vi "JKI-JSON Test Marshall-Unmarshall.vi"() -> ()   [LabVIEW 2019]
uses:
  Test Cluster.ctl
  <vilib>/addons/_JKI.lib/Serialization/JSON/Library/Timestamp Options.ctl
  source/Serializer.JSON.lvclass
  C:/Program Files (x86)/National Instruments/LabVIEW 2019/vi.lib/LabVIEW Open Source Project/OpenSerializer/Serializer/Serializer.lvclass
  source/Serializer.JSON.lvclass/Serializer.JSON.ctl
  source/Write Enums As String.vi
  source/Write Multiline.vi
  source/Write Numeric Extensions.vi
  source/Write Timestamp Options.vi
  <vilib>/LabVIEW Open Source Project/OpenSerializer/Serializer/Serializer.lvclass
  <vilib>/addons/_JKI.lib/Serialization/JSON/JKI JSON Serialization.lvlib
panel:
  in  "Timestamp Options":T1={"Convert Timestamps"=TRUE, "UTC"=FALSE}
  in  "Numeric Extensions":bool=TRUE
  in  "Multiline":bool=TRUE
  in  "Enums As String":bool=TRUE
  out "error out":errorcluster
  out "Pass?":bool
  out "Data Cluster out":T2={"Top-Level"={"Boolean"=FALSE, "String"="", "Path"=path "", "Numeric"=0.0, "Enum"=enum."Item0", "Array"=[], "Sub-Cluster"={"Numeric"=0.0, "Boolean"=FALSE, "Empty String"=""}, "Multi-Line String"=""}} {"Top-Level"."Numeric" format="%#_10g"}
  out "JSON String":string
  in  "Data Cluster in":T2={"Top-Level"={"Boolean"=FALSE, "String"="Another test string", "Path"=path "C:/Windows", "Numeric"=4.0, "Enum"=enum."Item0", "Array"=[0.0, 1.0, 2.0, 3.0, 4.0, 5.0, 6.0], "Sub-Cluster"={"Numeric"=0.0, "Boolean"=TRUE, "Empty String"="Test String Here"}, "Multi-Line String"="Test String Here\nLine2\nLine3"}} {"Top-Level"."Numeric" format="%#_10g"}
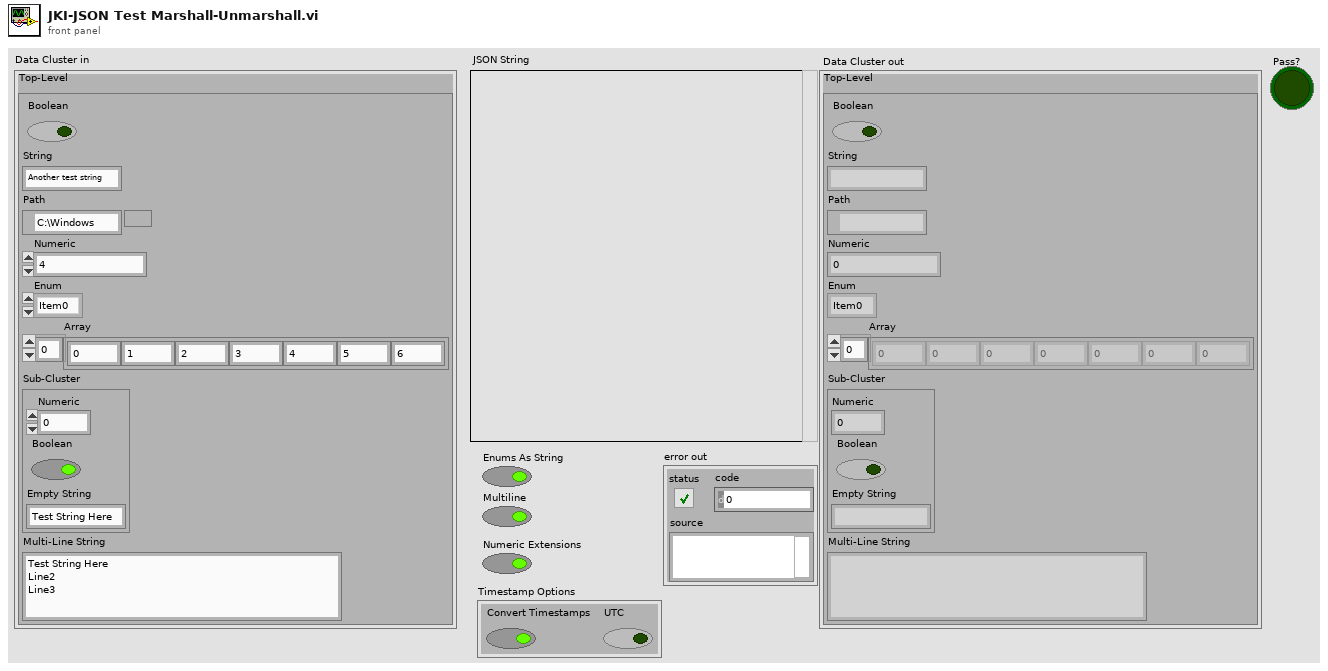
[diagram p1: front panel]
types:
  T1 = typedef "JKI JSON Serialization.lvlib/Timestamp Options.ctl" = cluster{"Convert Timestamps":bool, "UTC":bool}
  T2 = typedef "Test Cluster.ctl" = cluster{"Top-Level":cluster{"Boolean":bool, "String":string, "Path":path, "Numeric":dbl, "Enum":enum16{"Item0", "Item1"}, "Array":dbl[], "Sub-Cluster":cluster{"Numeric":dbl, "Boolean":bool, "Empty String":string}, "Multi-Line String":string}}
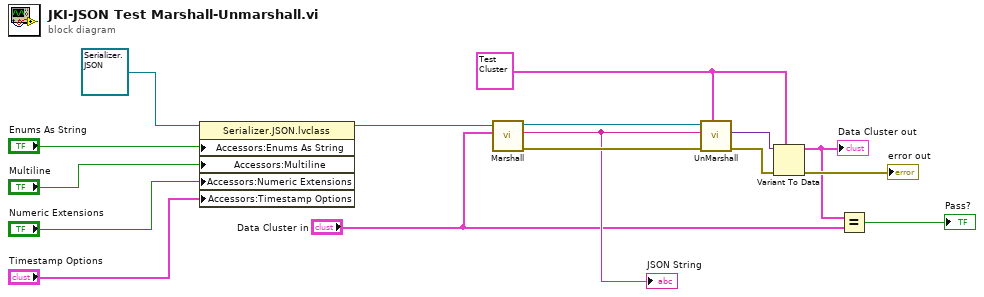
[diagram p0: block diagram]
diagram:
  w12 = T2 {"Top-Level"={"Boolean"=FALSE, "String"="", "Path"=path "", "Numeric"=0.0, "Enum"=enum."Item0", "Array"=[], "Sub-Cluster"={"Numeric"=0.0, "Boolean"=FALSE, "Empty String"=""}, "Multi-Line String"="Test String Here\nLine2\nLine3"}} ("Cluster")
  n1 = property class="Serializer.JSON.lvclass"(reference=refnum<class "Serializer.JSON.lvclass"> refnum ("OpenSerializer.JKI-JSON.lvlib:Serializer.JSON.lvclass"), "Accessors:Enums As String"="Enums As String", "Accessors:Multiline"="Multiline", "Accessors:Numeric Extensions"="Numeric Extensions", "Accessors:Timestamp Options"="Timestamp Options") -> (reference out=w8:refnum<class "Serializer.JSON.lvclass">)  [unwired: 1 in, 1 out]
  n2 = call <vilib>:"Marshall.vi"("Variant"="Data Cluster in", "Serializer in"=w8) -> ("error out"=w16:errorcluster, "String"=w11:string, "Serializer out"=w15:refnum<class "Serializer.JSON.lvclass">)  [unwired: 7 in]
  "JSON String" <- w11
  n3 = call <vilib>:"UnMarshall.vi"("Type"=w12, "error in (no error)"=w16, "String"=w11, "Serializer in"=w15) -> ("error out"=w14:errorcluster, "Variant"=w13:variant)  [unwired: 5 in, 1 out]
  n4 = Variant To Data(error in=w14, type=w12, Variant=w13) -> (data=w3:T2, error out=→"error out":errorcluster)
  "Data Cluster out" <- w3
  n5 = Equal?(x=w3, y="Data Cluster in") -> (x = y?=→"Pass?":bool)
